vi "Export Database Changes to CSV Files.vi"(10 "VS Filtered Change List":T1 {"Incoming"."Missing"."Node Ref" format="%.0x"; "Incoming"."Changed"."Old"."Node Ref" format="%.0x"; "Outgoing"."Missing"."Node Ref" format="%.0x"; "Outgoing"."Changed"."Old"."Node Ref" format="%.0x"}, 11 "Folder":path) -> (0 "error out":errorcluster)   [LabVIEW 2025, in "Protection and Counter Addon System Explorer.lvlib"]
uses:
  Protection and Counter Addon System Explorer.lvlib
  Types/Filtered XNET Changes.ctl
  Types/Database Changes.ctl
  Types/Base Frame Info_NoVS.ctl
  Types/Signal Attributes.ctl
  Types/CAN Filter Type.ctl
  Types/Base Frame Info.ctl
  <vilib>/NI VeriStand/Custom Device API/Custom Device Item Ref.ctl
  Types/Related CAN Frames.ctl
  Types/Related CAN Frames No VS.ctl
  <vilib>/NI VeriStand/Custom Device API/Custom Device API.lvlib
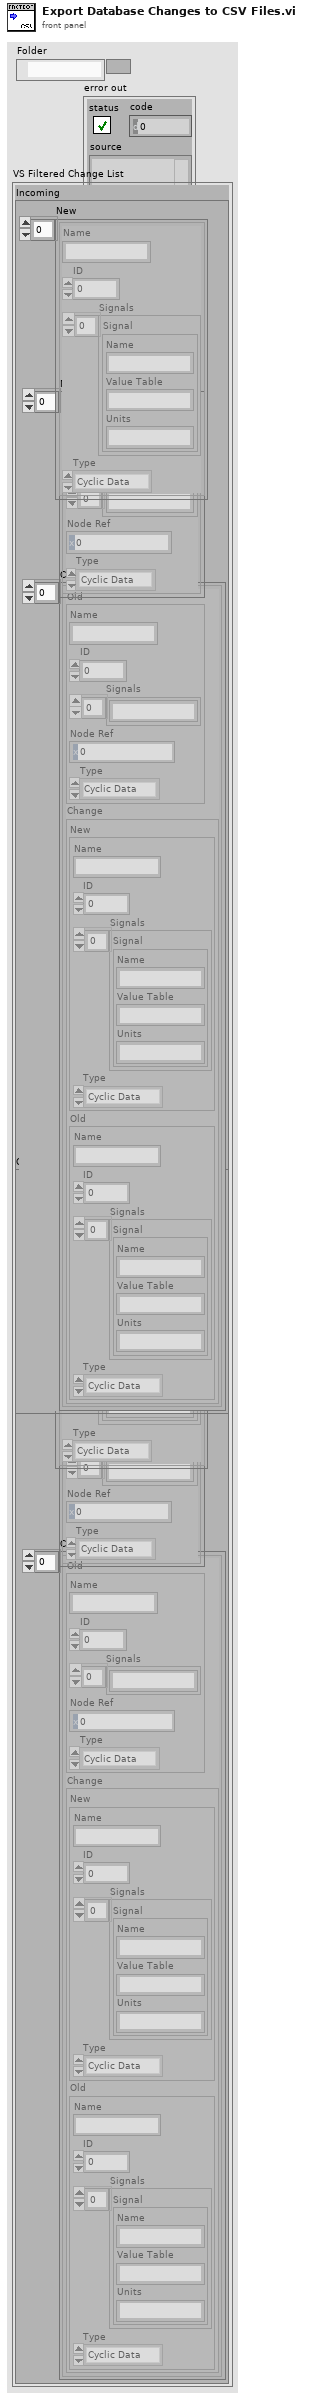
[diagram p1: front panel]
types:
  T1 = typedef "Protection and Counter Addon System Explorer.lvlib/Filtered XNET Changes.ctl" = cluster{"Incoming":T2, "Outgoing":T2}
  T2 = typedef "Protection and Counter Addon System Explorer.lvlib/Database Changes.ctl" = cluster{"New":T3[], "Missing":T6[], "Changed":T8[]}
  T3 = typedef "Protection and Counter Addon System Explorer.lvlib/Base Frame Info_NoVS.ctl" = cluster{"Name":string, "ID":u32, "Signals":T4[], "Type":T5}
  T4 = typedef "Protection and Counter Addon System Explorer.lvlib/Signal Attributes.ctl" = cluster{"Name":string, "Value Table":string, "Units":string}
  T5 = typedef "Protection and Counter Addon System Explorer.lvlib/CAN Filter Type.ctl" = enum16{"Cyclic Data", "Event Data", "Cyclic/Event", "All"}
  T6 = typedef "Protection and Counter Addon System Explorer.lvlib/Base Frame Info.ctl" = cluster{"Name":string, "ID":u32, "Signals":string[], "Node Ref":T7, "Type":T5}
  T7 = typedef "Custom Device API.lvlib/Custom Device Item Ref.ctl" = u64
  T8 = typedef "Protection and Counter Addon System Explorer.lvlib/Related CAN Frames.ctl" = cluster{"Old":T6, "Change":T9}
  T9 = typedef "Protection and Counter Addon System Explorer.lvlib/Related CAN Frames No VS.ctl" = cluster{"New":T3, "Old":T3}
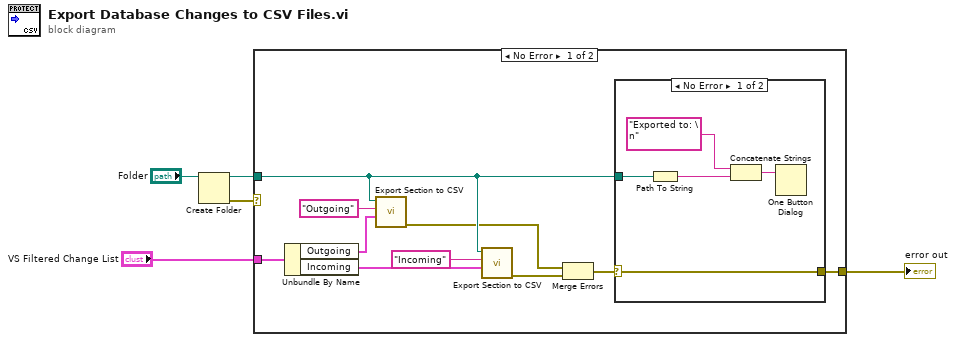
[diagram p0: block diagram]
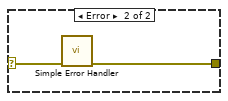
[diagram p2: hidden frame]
diagram:
  n1 = Create Folder(path (use dialog)="Folder") -> (created path=w4:path, error out=w3:errorcluster)  [unwired: 2 in, 1 out]
  n2 = case shown="No Error" w3 {
    selector: w3 -> [_ w23]
    tunnel: w4 -> [w10 _]
    tunnel: [w15 w23] -> w2
    tunnel: "VS Filtered Change List" -> [w14 _]
    frame No Error {
      n3 = Unbundle By Name(w14) -> ("Outgoing"=w13:T2, "Incoming"=w9:T2)
      n4 = call "Export Section to CSV.vi"("Database Changes"=w13, "Section"="Outgoing", "Folder"=w10) -> ("error out"=w8:errorcluster)  [unwired: 8 in]
      n5 = call "Export Section to CSV.vi"("Database Changes"=w9, "Section"="Incoming", "Folder"=w10) -> ("error out"=w7:errorcluster)  [unwired: 8 in]
      n6 = Merge Errors(w8, w7) -> (w6:errorcluster)
      n7 = case shown="No Error" w6 {
        selector: w6 -> [w20 w21]
        tunnel: [w20 w22] -> w15
        tunnel: w10 -> [w17 _]
        frame No Error {
          n8 = Path To String(path=w17) -> (string=w16:string)
          n9 = Concatenate Strings("Exported to: \n", w16) -> (w19:string)
          n10 = One Button Dialog(message=w19) -> ()  [unwired: 1 in, 1 out]
        }
        frame Error {
          n11 = call <vilib>:"Simple Error Handler.vi"("error in (no error)"=w21) -> ("error out"=w22:errorcluster)  [unwired: 4 in, 4 out]
        }
      }
    }
    frame Error {
    }
  }
  "error out" <- w2
